vi "Sys config window-Set wavelengths ring.vi"(9 "Laser wavelength (nm)":u16, 11 "System Config window refs":T1) -> (1 "Wavelength already exists":bool)   [LabVIEW 2013]
uses:
  Typedefs/HW config window refs cluster.ctl
  Typedefs/HW Setup tab control.ctl
  Typedefs/DAQ FPGA config cluster.ctl
  RIG-SPECIFIC FILES/FPGA Refs/FPGA Ref.ctl
  <vilib>/userdefined/High Color/nirio_resource_hc.ctl
  Typedefs/FPGA input type AC-DC.ctl
  Peripherals Control/Triggers/Typedefs/Triggers output setup.ctl
  Peripherals Control/Triggers/Typedefs/Trigger setup element cluster.ctl
  Typedefs/AOL Properties Cluster.ctl
  Typedefs/CTRL system config cluster ref.ctl
  Typedefs/CTRL system config cluster.ctl
  Configuration code/Calibration/Globals/gl_Calibration globals.vi
panel:
  # "<----Typedef"
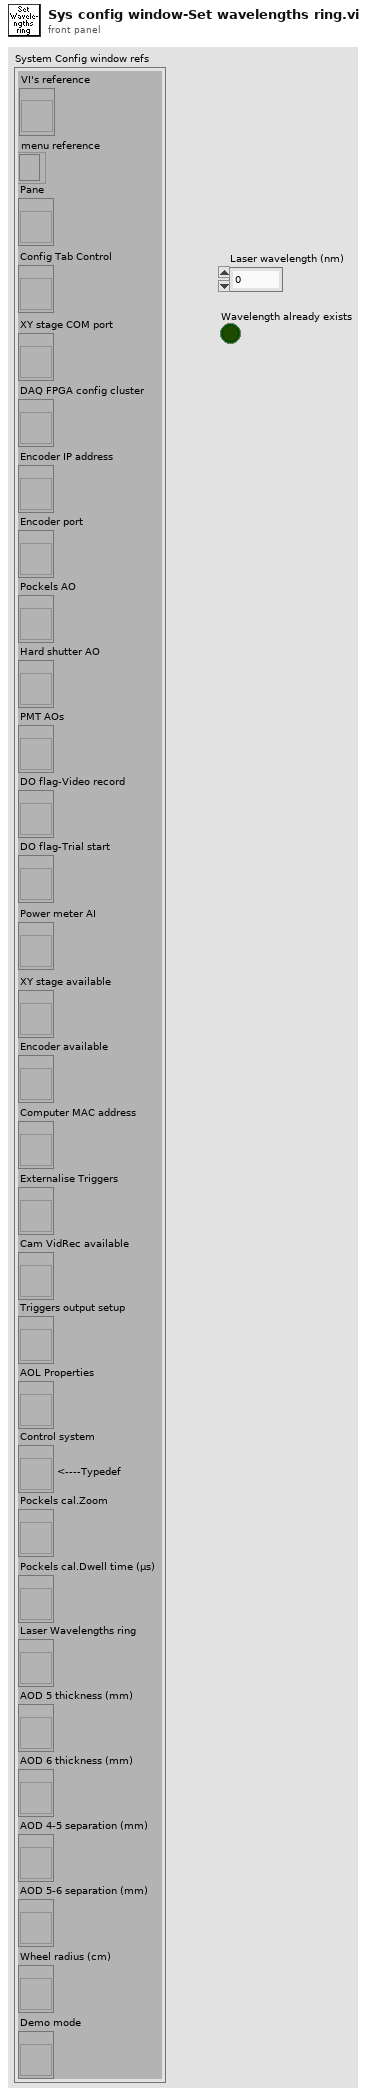
[diagram p1: front panel]
types:
  T1 = typedef "HW config window refs cluster.ctl" = cluster{"VI's reference":refnum<vi>, "menu reference":refnum<k9>, "Pane":refnum<vi>, "Config Tab Control":refnum<vi>, "XY stage COM port":refnum<vi>, "DAQ FPGA config cluster":refnum<vi>, "Encoder IP address":refnum<vi>, "Encoder port":refnum<vi>, "Pockels AO":refnum<vi>, "Hard shutter AO":refnum<vi>, "PMT AOs":refnum<vi>, "DO flag-Video record":refnum<vi>, "DO flag-Trial start":refnum<vi>, "Power meter AI":refnum<vi>, "XY stage available":refnum<vi>, "Encoder available":refnum<vi>, "Computer MAC address":refnum<vi>, "Externalise Triggers":refnum<vi>, "Cam VidRec available":refnum<vi>, "Triggers output setup":refnum<vi>, "AOL Properties":refnum<vi>, "Control system":T2, "Pockels cal.Zoom":refnum<vi>, "Pockels cal.Dwell time (µs)":refnum<vi>, "Laser Wavelengths ring":refnum<vi>, "AOD 5 thickness (mm)":refnum<vi>, "AOD 6 thickness (mm)":refnum<vi>, "AOD 4-5 separation (mm)":refnum<vi>, "AOD 5-6 separation (mm)":refnum<vi>, "Wheel radius (cm)":refnum<vi>, "Demo mode":refnum<vi>}
  T2 = typedef "CTRL system config cluster ref.ctl" = refnum<vi>
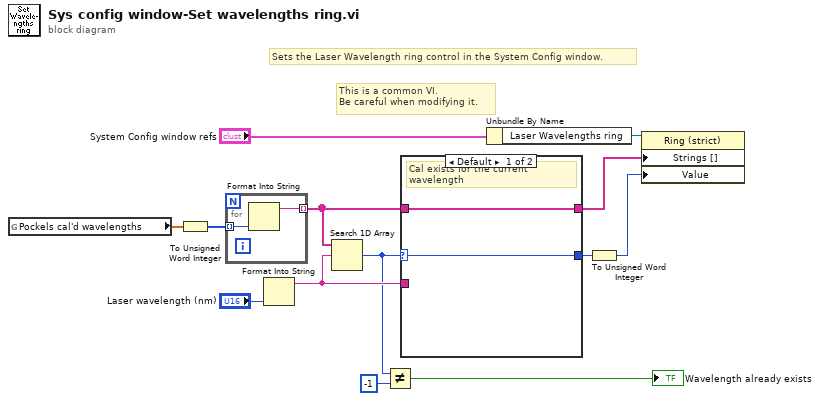
[diagram p0: block diagram]
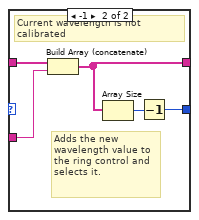
[diagram p2: hidden frame]
diagram:
  # "This is a common VI.\nBe careful when modifying it."
  # "Sets the Laser Wavelength ring control in the System Config window."
  n1 = global read "gl_Calibration globals.vi" "Pockels cal'd wavelengths"() -> (w12:dbl[])
  n2 = To Unsigned Word Integer(number=w12) -> (unsigned 16bit integer=w11:u16[])
  n3 = for {
    tunnel: w11 -> [w15] mode=indexing
    tunnel: [w14] -> w4 mode=indexing
    n4 = Format Into String(w15) -> (resulting string=w14:string)  [unwired: 3 in, 1 out]
  }
  n5 = Format Into String("Laser wavelength (nm)") -> (resulting string=w5:string)  [unwired: 3 in, 1 out]
  n6 = Search 1D Array(1D array=w4, element=w5) -> (index of element=w3:i32)  [unwired: 1 in]
  n7 = Not Equal?(x=w3, y=-1) -> (x != y?=→"Wavelength already exists":bool)
  n8 = case shown="Default" w3 {
    selector: w3 -> [w17 _]
    tunnel: [w17 w18] -> w8
    tunnel: w4 -> [w16 w21]
    tunnel: w5 -> [_ w22]
    tunnel: [w16 w20] -> w6
    frame Default {
      # "Cal exists for the current wavelength"
    }
    frame -1 {
      # "Adds the new wavelength value to the ring control and selects it."
      # "Current wavelength is not calibrated"
      n9 = Build Array (concatenate)(w21, w22) -> (w20:string[])
      n10 = Array Size(array=w20) -> (size(s)=w19:i32)
      n11 = Decrement(x=w19) -> (x-1=w18:i32)
    }
  }
  n12 = Unbundle By Name("System Config window refs") -> ("Laser Wavelengths ring"=w7:refnum<vi>)
  n13 = To Unsigned Word Integer(number=w8) -> (unsigned 16bit integer=w9:u16)
  n14 = property on="Property Node" class="Ring (strict)"(reference=w7, "Strings []"=w6, "Value"=w9) -> ()  [unwired: 1 in, 2 out]
